vi "set_voltage.vi"(1 "Voltage":dbl min=0.0 max=5.0, 2 "Channel Index":i32=1 min=1 max=4, 3 "Slot":i32=4 min=0 max=14, 4 "69321B?":bool) -> ()   [LabVIEW 2011]
uses:
  globals.vi
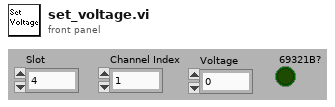
[diagram p1: front panel]
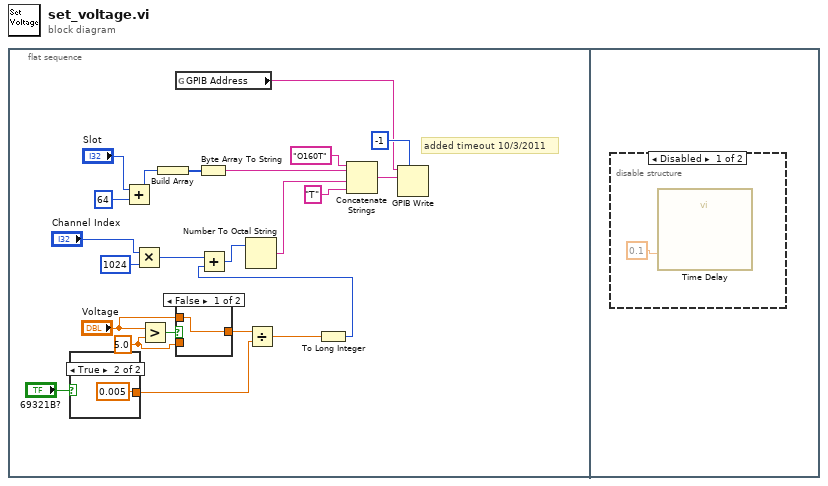
[diagram p0: block diagram]
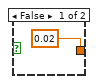
[diagram p3: hidden frame]
diagram:
  n1 = flat-sequence {
    frame #0 {
      w15 = 5.0 ("y")
      # "added timeout 10/3/2011"
      n2 = case shown="True" "69321B?" {
        tunnel: [0.02 ("y") 0.005 ("y")] -> w8
        frame False {
        }
        frame True {
        }
      }
      n3 = Add(x="Slot", y=u32 64) -> (x+y=w4:u32)
      n4 = Multiply(x="Channel Index", y=1024) -> (x*y=w21:i32)
      n5 = Greater?(x="Voltage", y=w15) -> (0:w14:bool)
      n6 = Build Array(w4) -> (w3:u32[])
      n7 = global read "globals.vi" "GPIB Address"() -> (w19:string)
      n8 = case shown="False" w14 {
        tunnel: w15 -> [_ w25]
        tunnel: [w24 w25] -> w16
        tunnel: "Voltage" -> [w24 _]
        frame False {
        }
        frame True {
        }
      }
      n9 = Byte Array To String(unsigned byte array=w3) -> (string=w11:string)
      n10 = Divide(x=w16, y=w8) -> (x/y=w20:dbl)
      n11 = To Long Integer(number=w20) -> (32bit integer=w9:i32)
      n12 = Add(x=w21, y=w9) -> (x+y=w12:i32)
      n13 = Number To Octal String(2:w12) -> (0:w13:string)  [unwired: 1 out]
      n14 = Concatenate Strings("O160T" ("string"), w11, w13, "T" ("string")) -> (w7:string)
      n15 = GPIB Write(0:w19, 1:w7, 4:-1 ("timeout ms (488.2 global)")) -> ()  [unwired: 1 in, 3 out]
    }
    frame #1 {
      n16 = disable-structure shown="Disabled" {
        frame Disabled {
          n17 = call "Time Delay"("Delay Time (s)"=0.1) -> ()  [unwired: 1 in, 10 out]
        }
        frame Enabled {
        }
      }
    }
  }
